vi "PRIME Telescope Offset Commands.vi"(8 "error in (no error)":errorcluster, 10 "Offsets":T1, 11 "connection ID":refnum<k5>) -> (0 "error out":errorcluster, 3 "connection ID dup":refnum<k5>)   [LabVIEW 2024, in "PRIME Telescope.lvclass"]
uses:
  PRIME Telescope.lvclass
  CC cluster Telescope Offsets.ctl
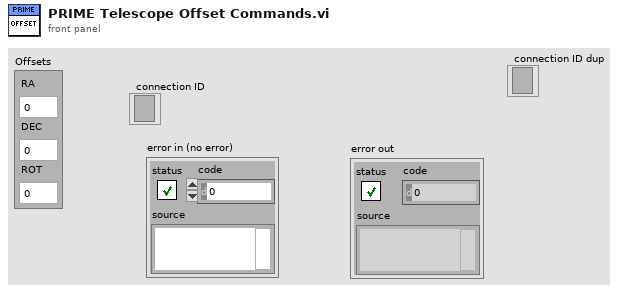
[diagram p1: front panel]
types:
  T1 = typedef "CC cluster Telescope Offsets.ctl" = cluster{"RA":dbl, "DEC":dbl, "ROT":dbl}
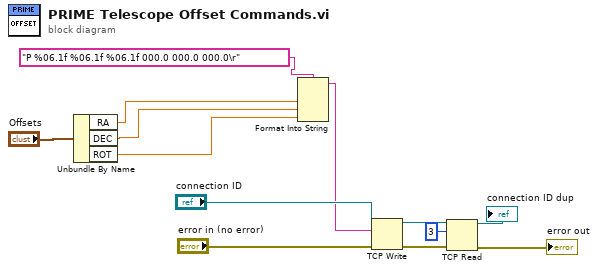
[diagram p0: block diagram]
diagram:
  n1 = Unbundle By Name("Offsets") -> ("RA"=w6:dbl, "DEC"=w5:dbl, "ROT"=w4:dbl)
  n2 = Format Into String(format string="P %06.1f %06.1f %06.1f 000.0 000.0 000.0\r", w6, w5, w4) -> (resulting string=w2:string)  [unwired: 2 in, 1 out]
  n3 = TCP Write(connection ID="connection ID", data in=w2, error in (no error)="error in (no error)") -> (connection ID out=w10:refnum<k5>, error out=w11:errorcluster)  [unwired: 1 in, 1 out]
  n4 = TCP Read(connection ID=w10, bytes to read=3, error in (no error)=w11) -> (connection ID out=→"connection ID dup":refnum<k5>, error out=→"error out":errorcluster)  [unwired: 2 in, 1 out]
